vi "Get Children.vi"(8 "error in (no error)":errorcluster, 11 "Attribute in":refnum<class "Attribute.lvclass">) -> (0 "error out":errorcluster, 2 "Children":refnum<class "Data Item.lvclass">[](array[class]), 3 "Attribute out":refnum<class "Attribute.lvclass">)   [LabVIEW 2018, in "VILab.lvlib" / "Attribute.lvclass"]
uses:
  Attribute.lvclass
  Data Item.lvclass
  Attribute.lvclass/Attribute.ctl
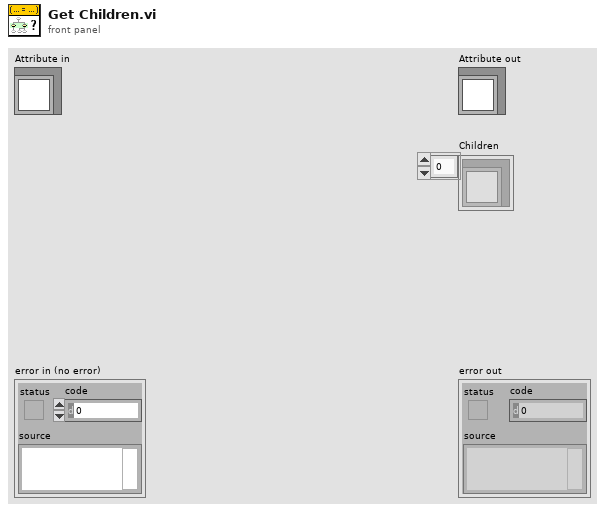
[diagram p1: front panel]
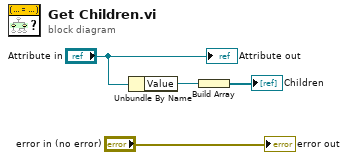
[diagram p0: block diagram]
diagram:
  n1 = Unbundle By Name("Attribute in") -> ("Value"=w2:refnum<class "Data Item.lvclass">)
  n2 = Build Array(w2) -> (→"Children":refnum<class "Data Item.lvclass">[])
  "error out" <- "error in (no error)"
  "Attribute out" <- "Attribute in"
